vi "Serialize - JSON.vi"(8 "error in":errorcluster, 11 "Alicat Data in":refnum<class "Alicat Data.lvclass">) -> (0 "error out":errorcluster, 2 "Serialized JSON":string, 3 "Alicat Data out":refnum<class "Alicat Data.lvclass">)   [LabVIEW 2015, in "Alicat Lib.lvlib" / "Alicat Data.lvclass"]
uses:
  Alicat Data.lvclass
  <vilib>/MSR Consulting, LLC/General Reuse/Data/Data.lvclass/Data.ctl
  Alicat Data.lvclass/Alicat Data.ctl
  <vilib>/MSR Consulting, LLC/General Reuse/Data/Read Data ID.vi
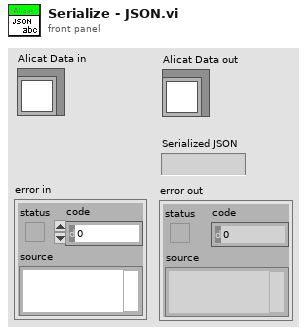
[diagram p1: front panel]
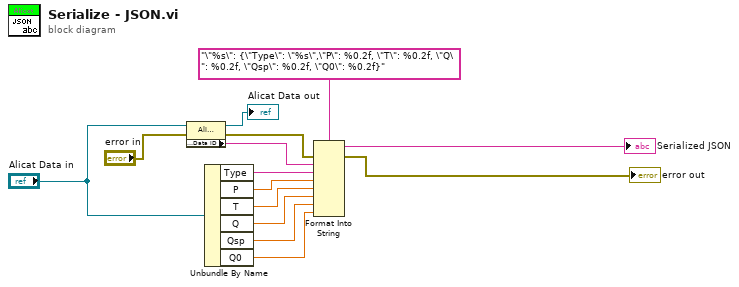
[diagram p0: block diagram]
diagram:
  n1 = property class="Alicat Data"(reference="Alicat Data in", error in="error in") -> (reference out=→"Alicat Data out":refnum<class "Alicat Data.lvclass">, error out=w2:errorcluster, "Accessors:Data ID"=w4:string)
  n2 = Unbundle By Name("Alicat Data in") -> ("Type"=w12:string, "P"=w11:sgl, "T"=w10:sgl, "Q"=w9:sgl, "Qsp"=w8:sgl, "Q0"=w7:sgl)
  n3 = Format Into String(format string="\"%s\": {\"Type\": \"%s\",\"P\": %0.2f, \"T\": %0.2f, \"Q\": %0.2f, \"Qsp\": %0.2f, \"Q0\": %0.2f}" ("string"), error in=w2, w4, w12, w11, w10, w9, w8, w7) -> (resulting string=→"Serialized JSON":string, error out=→"error out":errorcluster)  [unwired: 1 in]
